vi "Set Parameters Configuration File Path.vi"(8 "error in":errorcluster, 9 "parameters configuration file path":path, 11 "Ballard ARINC 429 custom device in":T1 format="%.0x") -> (0 "error out":errorcluster, 3 "Ballard ARINC 429 custom device out":T1 format="%.0x")   [LabVIEW 2020, in "Ballard ARINC 429 Scripting.lvlib"]
doc: "Specifies the <b>parameters configuration file path</b>. The parameters configuration file is not deployed to the RT target, but it must be consistent with the hardware configuration for successful deployment and avionics bus communication."
uses:
  Ballard ARINC 429 Scripting.lvlib
  <vilib>/NI VeriStand/Custom Device API/Custom Device Item Ref.ctl
  Constants.vi
  <vilib>/NI VeriStand/Custom Device API/Set Item Property (Dependent File).vi
  <vilib>/NI VeriStand/Custom Device API/Custom Device API.lvlib
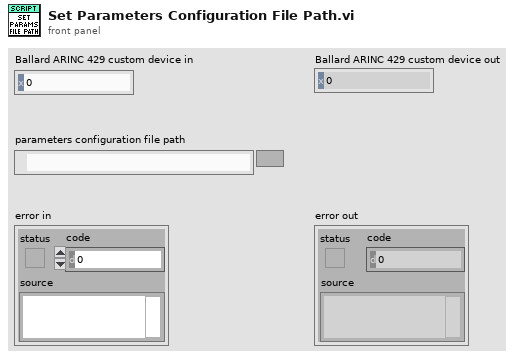
[diagram p1: front panel]
types:
  T1 = typedef "Custom Device API.lvlib/Custom Device Item Ref.ctl" = u64
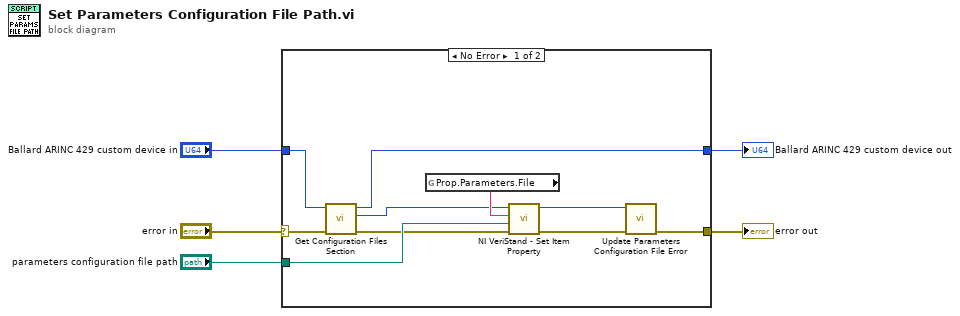
[diagram p0: block diagram]
diagram:
  n1 = case shown="No Error" "error in" {
    selector: "error in" -> [w10 w17]
    tunnel: "Ballard ARINC 429 custom device in" -> [w7 w16]
    tunnel: [w11 w17] -> w4
    tunnel: "parameters configuration file path" -> [w15 _]
    tunnel: [w6 w16] -> w1
    frame No Error {
      n2 = call "Get Configuration Files Section.vi"("error in"=w10, "Custom device Ref"=w7) -> ("error out"=w9:errorcluster, "Configuration files Ref"=w8:T1, "Custom device Ref out"=w6:T1)  [unwired: 7 in]
      n3 = global read "Constants.vi" "Prop.Parameters.File"() -> (w14:string)
      n4 = call-poly <vilib>:"NI VeriStand - Set Item Property.vi"("error in (no error)"=w9, "Path"=w15, "Property Name"=w14, "Item Ref in"=w8) -> ("error out"=w12:errorcluster, "Item Ref out"=w13:T1)  [unwired: 5 in, 1 out]
      n5 = call "Update Parameters Configuration File Error.vi"("error in"=w12, "Configuration files Ref"=w13) -> ("error out"=w11:errorcluster)  [unwired: 8 in, 1 out]
    }
    frame Error {
    }
  }
  "error out" <- w4
  "Ballard ARINC 429 custom device out" <- w1
